vi "libssh2_channel_eof.vi"(8 "error in (no error)":errorcluster, 11 "channel":T1) -> (0 "error out":errorcluster, 3 "return value":i32)   [LabVIEW 2013, in "libssh2.lvlib"]
doc: "Checks if the remote host has sent an EOF status for the channel."
uses:
  libssh2.lvlib
  Channel Refnum.ctl
  libssh2.dll
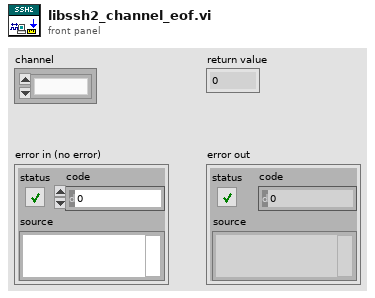
[diagram p1: front panel]
types:
  T1 = typedef "libssh2.lvlib/Channel Refnum.ctl" = refnum<k1>
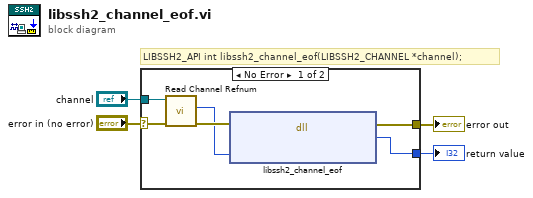
[diagram p0: block diagram]
diagram:
  # "LIBSSH2_API int libssh2_channel_eof(LIBSSH2_CHANNEL *channel);"
  n1 = case shown="No Error" "error in (no error)" {
    selector: "error in (no error)" -> [w5 w11]
    tunnel: [w10 _] -> w4
    tunnel: [w9 w11] -> w3
    tunnel: "channel" -> [w6 _]
    frame No Error {
      n2 = call "Read Channel Refnum.vi"("error in (no error)"=w5, "channel"=w6) -> ("error out"=w8:errorcluster, "LIBSSH2_CHANNEL*"=w7:u64)  [unwired: 8 in]
      n3 = dll-call lib="C:/Users/pasca/source/repos/libssh2-labview/libssh2**.*" fn="libssh2_channel_eof"(error in=w8, "channel"=w7) -> (error out=w9:errorcluster, "return value"=w10:i32)  [unwired: 3 in, 1 out]
    }
    frame Error {
    }
  }
  "return value" <- w4
  "error out" <- w3
